vi "GetProperties.vi"(8 "error in":errorcluster, 11 "SubVI in":refnum<class "SubVI.lvclass">) -> (0 "error out":errorcluster, 3 "SubVI out":refnum<class "SubVI.lvclass">)   [LabVIEW 2014, in "SubVI.lvclass"]
uses:
  SubVI.lvclass
  SubVI.lvclass/SubVI.ctl
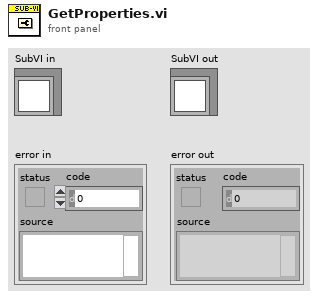
[diagram p1: front panel]
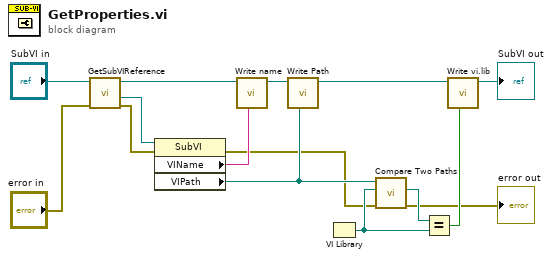
[diagram p0: block diagram]
diagram:
  n1 = call "GetSubVIReference.vi"("error in"="error in", "SubVI in"="SubVI in") -> ("error out"=w12:errorcluster, "SubVI reference"=w13:refnum<vi>, "SubVI out"=w11:refnum<class "SubVI.lvclass">)  [unwired: 7 in]
  n2 = property class="SubVI"(reference=w13, error in=w12) -> (error out=w5:errorcluster, "VIName"=w10:string, "VIPath"=w6:path)  [unwired: 1 out]
  n3 = call-dynamic "Write name.vi"("name"=w10, "Node in"=w11) -> ("Node out"=w9:refnum<class "SubVI.lvclass">)  [unwired: 7 in]
  n4 = call "Write Path.vi"("Path"=w6, "SubVI in"=w9) -> ("SubVI out"=w4:refnum<class "SubVI.lvclass">)  [unwired: 7 in]
  n5 = VI Library() -> (path=w7:path)
  n6 = call <vilib>:"Compare Two Paths.vi"("error in (no error)"=w5, "Path 2"=w7, "Path 1"=w6) -> ("error out"=→"error out":errorcluster, "Common Path"=w8:path)  [unwired: 5 in, 2 out]
  n7 = Equal?(x=w8, y=w7) -> (x = y?=w3:bool)
  n8 = call "Write vi.lib.vi"("vi.lib"=w3, "SubVI in"=w4) -> ("SubVI out"=→"SubVI out":refnum<class "SubVI.lvclass">)  [unwired: 7 in]
